vi "References FGV.vi"(7 "Ref Action":T2, 8 "error in":errorcluster, 11 "References In":T1) -> (0 "error out":errorcluster, 3 "References Out":T1)   [LabVIEW 2024, in "Tester InterComm.lvlib"]
uses:
  Tester InterComm.lvlib
  General Actions.ctl
  Type Definitions/Tester References.ctl
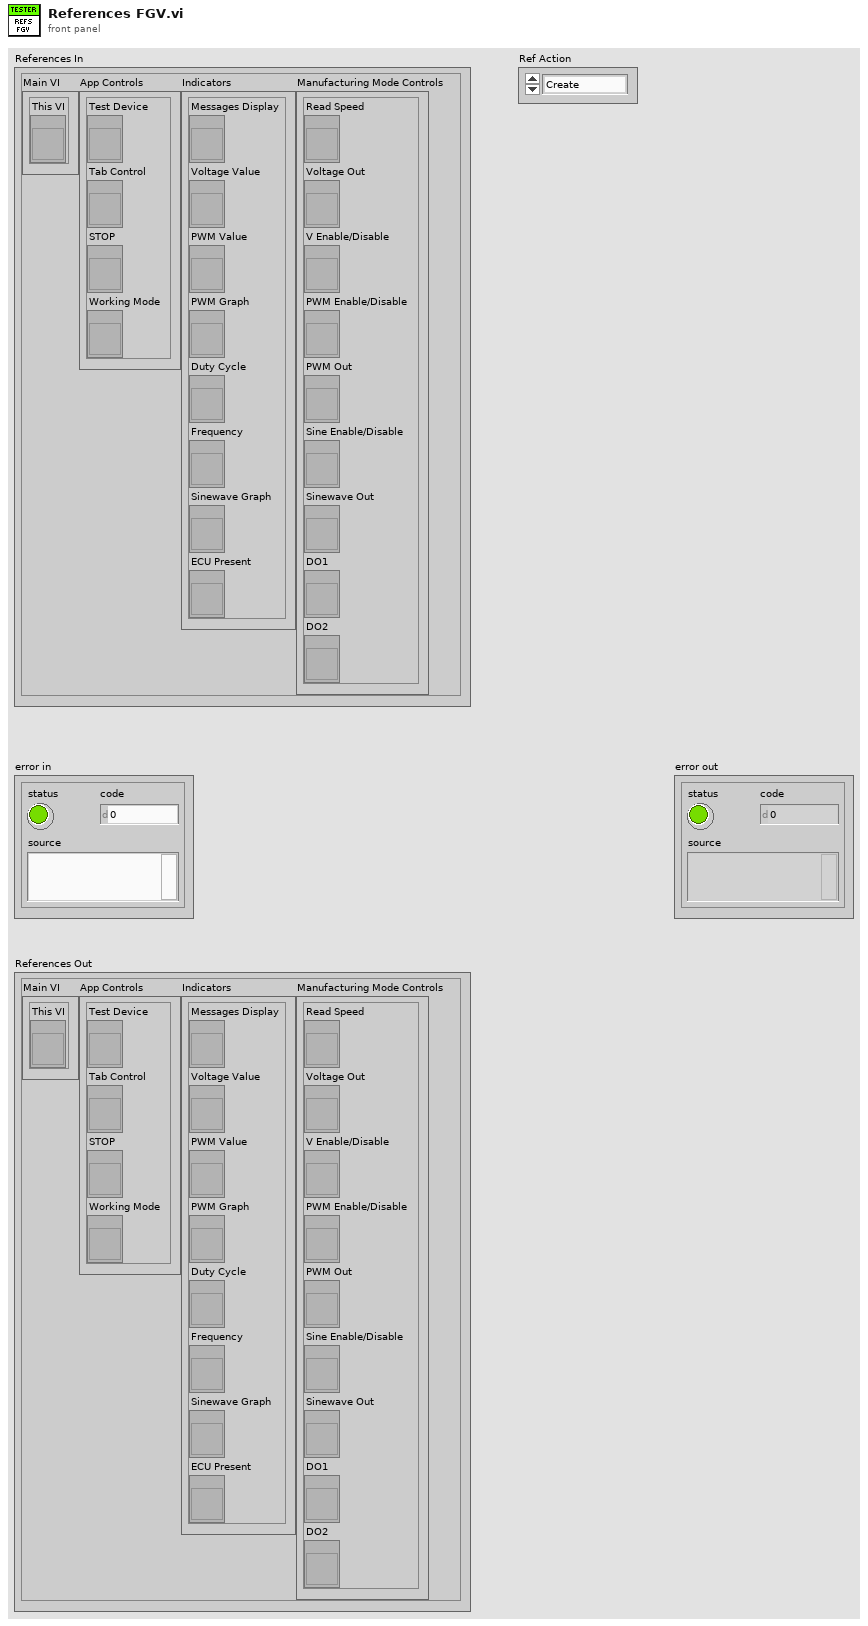
[diagram p1: front panel]
types:
  T1 = typedef "Tester InterComm.lvlib/Tester References.ctl" = cluster{"Main VI":cluster{"This VI":refnum<vi>}, "App Controls":cluster{"Test Device":refnum<vi>, "Tab Control":refnum<vi>, "STOP":refnum<vi>, "Working Mode":refnum<vi>}, "Indicators":cluster{"Messages Display":refnum<vi>, "Voltage Value":refnum<vi>, "PWM Value":refnum<vi>, "PWM Graph":refnum<vi>, "Duty Cycle":refnum<vi>, "Frequency":refnum<vi>, "Sinewave Graph":refnum<vi>, "ECU Present":refnum<vi>}, "Manufacturing Mode Controls":cluster{"Read Speed":refnum<vi>, "Voltage Out":refnum<vi>, "V Enable/Disable":refnum<vi>, "PWM Enable/Disable":refnum<vi>, "PWM Out":refnum<vi>, "Sine Enable/Disable":refnum<vi>, "Sinewave Out":refnum<vi>, "DO1":refnum<vi>, "DO2":refnum<vi>}}
  T2 = typedef "Tester InterComm.lvlib/General Actions.ctl" = enum16{"Create", "Get", "Destroy"}
  T3 = cluster{"Test Device":refnum<vi>, "Tab Control":refnum<vi>, "STOP":refnum<vi>, "Working Mode":refnum<vi>}
  T4 = cluster{"Messages Display":refnum<vi>, "Voltage Value":refnum<vi>, "PWM Value":refnum<vi>, "PWM Graph":refnum<vi>, "Duty Cycle":refnum<vi>, "Frequency":refnum<vi>, "Sinewave Graph":refnum<vi>, "ECU Present":refnum<vi>}
  T5 = cluster{"Read Speed":refnum<vi>, "Voltage Out":refnum<vi>, "V Enable/Disable":refnum<vi>, "PWM Enable/Disable":refnum<vi>, "PWM Out":refnum<vi>, "Sine Enable/Disable":refnum<vi>, "Sinewave Out":refnum<vi>, "DO1":refnum<vi>, "DO2":refnum<vi>}
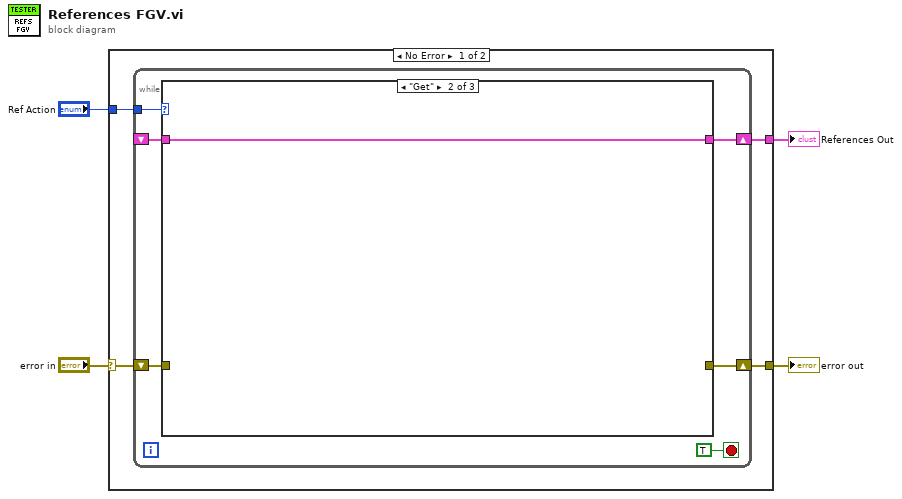
[diagram p0: block diagram]
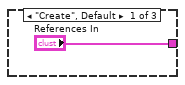
[diagram p2: hidden frame]
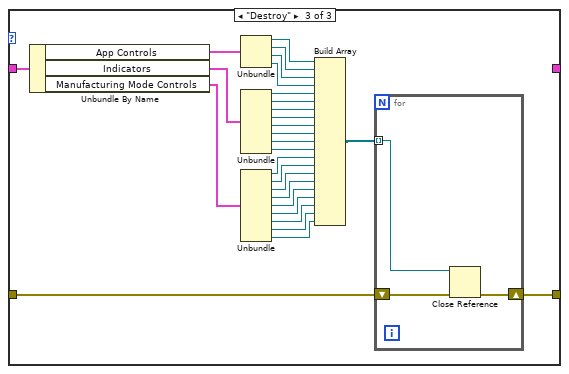
[diagram p3: hidden frame]
diagram:
  n1 = case shown="No Error" "error in" {
    selector: "error in" -> [w5 w48]
    tunnel: "Ref Action" -> [w8 _]
    tunnel: [w7 _] -> w3
    tunnel: [w6 w48] -> w2
    frame No Error {
      n2 = while {
        tunnel: w8 -> [w13]
        shift-right: [w12] -> w7
        shift-left: _ -> [w11]
        shift-right: [w10] -> w6
        shift-left: w5 -> [w9]
        stop <- TRUE stop-if-true
        n3 = case shown="\"Get\"" w13 {
          tunnel: ["References In" w16 _] -> w12
          tunnel: w11 -> [_ w16 w44]
          tunnel: [_ _ w19] -> w10
          tunnel: w9 -> [_ _ w17]
          frame "Create", Default {
          }
          frame "Get" {
          }
          frame "Destroy" {
            n4 = Unbundle By Name(w44) -> ("App Controls"=w43:T3, "Indicators"=w42:T4, "Manufacturing Mode Controls"=w41:T5)
            n5 = Unbundle(w43) -> ("Test Device"=w40:refnum<vi>, "Tab Control"=w39:refnum<vi>, "STOP"=w38:refnum<vi>, "Working Mode"=w37:refnum<vi>)
            n6 = Unbundle(w42) -> ("Messages Display"=w36:refnum<vi>, "Voltage Value"=w35:refnum<vi>, "PWM Value"=w34:refnum<vi>, "PWM Graph"=w33:refnum<vi>, "Duty Cycle"=w32:refnum<vi>, "Frequency"=w31:refnum<vi>, "Sinewave Graph"=w30:refnum<vi>, "ECU Present"=w29:refnum<vi>)
            n7 = Unbundle(w41) -> ("Read Speed"=w28:refnum<vi>, "Voltage Out"=w27:refnum<vi>, "V Enable/Disable"=w26:refnum<vi>, "PWM Enable/Disable"=w25:refnum<vi>, "PWM Out"=w24:refnum<vi>, "Sine Enable/Disable"=w23:refnum<vi>, "Sinewave Out"=w22:refnum<vi>, "DO1"=w21:refnum<vi>, "DO2"=w20:refnum<vi>)
            n8 = Build Array(w40, w39, w38, w37, w36, w35, w34, w33, w32, w31, w30, w29, w28, w27, w26, w25, w24, w23, w22, w21, w20) -> (w18:refnum<vi>[])
            n9 = for {
              shift-right: [w47] -> w19
              shift-left: w17 -> [w46]
              tunnel: w18 -> [w45] mode=indexing
              n10 = Close Reference(reference=w45, error in (no error)=w46) -> (error out=w47:errorcluster)
            }
          }
        }
      }
    }
    frame Error {
    }
  }
  "References Out" <- w3
  "error out" <- w2
